vi "Move to Abs Step location.vi"(8 "error in (no error)":errorcluster, 10 "Absolute step location to move":i32, 11 "Lifter_motor in":refnum<class "Lifter_motor.lvclass">) -> (0 "error out":errorcluster, 2 "Driver ACK?":bool, 3 "Lifter_motor out":refnum<class "Lifter_motor.lvclass">)   [LabVIEW 2019, in "Lifter_motor.lvclass"]
uses:
  Lifter_motor.lvclass
  Lifter_motor.lvclass/Lifter_motor.ctl
  TCP Class/LifterTCP.lvclass
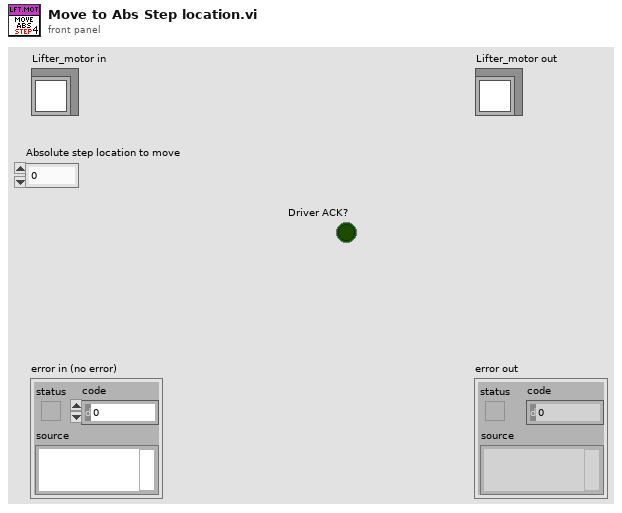
[diagram p1: front panel]
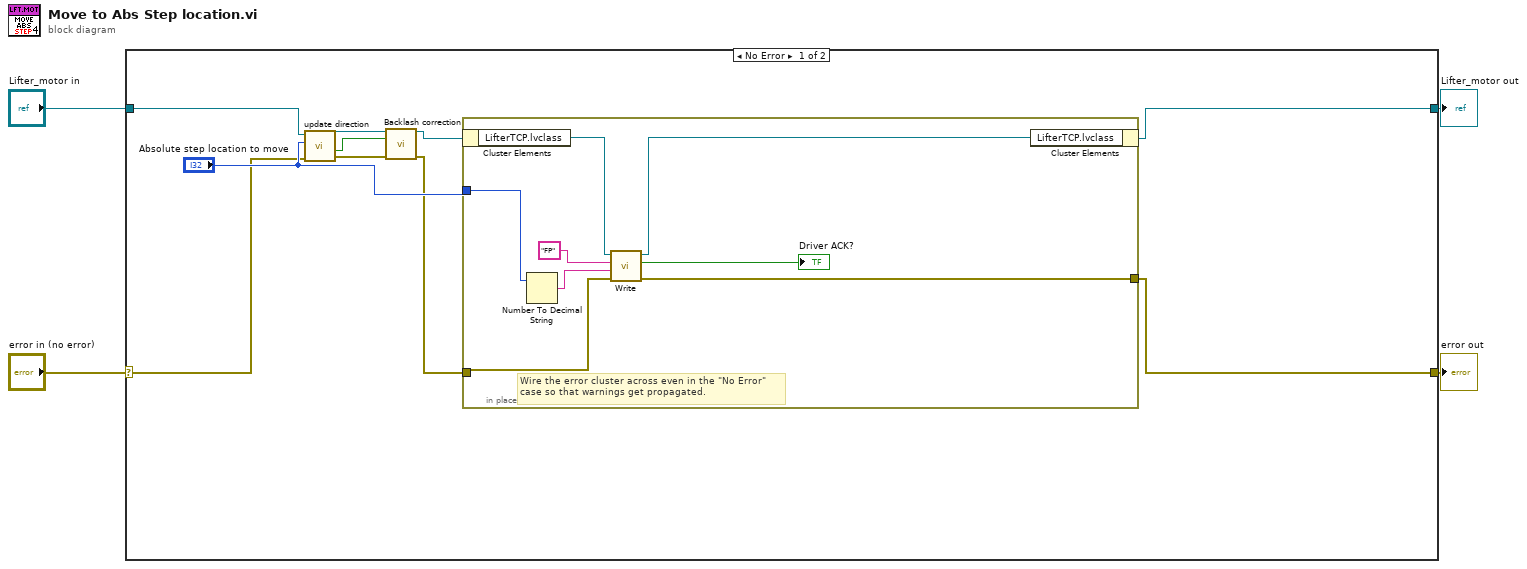
[diagram p0: block diagram]
diagram:
  n1 = case shown="No Error" "error in (no error)" {
    selector: "error in (no error)" -> [w11 w24]
    tunnel: [w13 w24] -> w3
    tunnel: [w14 w23] -> w1
    tunnel: "Lifter_motor in" -> [w10 w23]
    frame No Error {
      n2 = call "update direction.vi"("error in (no error)"=w11, "Absolute step location to move"="Absolute step location to move", "Lifter_motor in"=w10) -> ("error out"=w5:errorcluster, "Direction changed"=w7:bool, "Lifter_motor out"=w8:refnum<class "Lifter_motor.lvclass">)  [unwired: 5 in, 1 out]
      n3 = call "Backlash correction.vi"("Lifter_motor in"=w8, "Direction is chaged"=w7, "error in (no error)"=w5) -> ("Lifter_motor out"=w9:refnum<class "Lifter_motor.lvclass">, "error out"=w6:errorcluster)  [unwired: 11 in]
      n4 = in-place {
        in-place-border: [w19] -> w13
        in-place-border: "Absolute step location to move" -> [w16]
        in-place-border: w6 -> [w15]
        # "Wire the error cluster across even in the \"No Error\"\ncase so that warnings get propagated."
        n5 = in-place-cluster #1(w9) -> ("LifterTCP.lvclass"=w20:refnum<class "LifterTCP.lvclass">)
        n6 = Number To Decimal String(number=w16) -> (decimal integer string=w22:string)  [unwired: 1 in]
        n7 = call "Write.vi"("error in (no error)"=w15, "Parameter 2"=w22, "Parameter 1"="FP" ("string"), "LifterTCP in"=w20) -> ("error out"=w19:errorcluster, "Driver ACK?"=→"Driver ACK?":bool, "LifterTCP out"=w17:refnum<class "LifterTCP.lvclass">)  [unwired: 5 in]
        n8 = in-place-cluster #1("LifterTCP.lvclass"=w17) -> (w14:refnum<class "Lifter_motor.lvclass">)
      }
    }
    frame Error {
    }
  }
  "error out" <- w3
  "Lifter_motor out" <- w1
